vi "Functaion Air Temperature to Density.vi"(5 "Temp(F)":dbl) -> (6 "Density (lb/ft3)":dbl)   [LabVIEW 2012]
uses:
  <vilib>/gmath/NI_Gmath.lvlib
panel:
  in  "Density":dbl[](array[numeric])=[0.081, 0.08, 0.0766, 0.073, 0.0717, 0.071, 0.0698, 0.0692, 0.0685, 0.0674, 0.0662, 0.0651, 0.064, 0.063, 0.062, 0.061, 0.0601, 0.0592, 0.057, 0.055, 0.0531, 0.0513]
  in  "Temps":dbl[](array[numeric])=[30.0, 40.0, 50.0, 75.0, 85.0, 95.0, 100.0, 105.0, 110.0, 120.0, 130.0, 140.0, 150.0, 160.0, 170.0, 180.0, 190.0, 200.0, 225.0, 250.0, 275.0, 300.0]
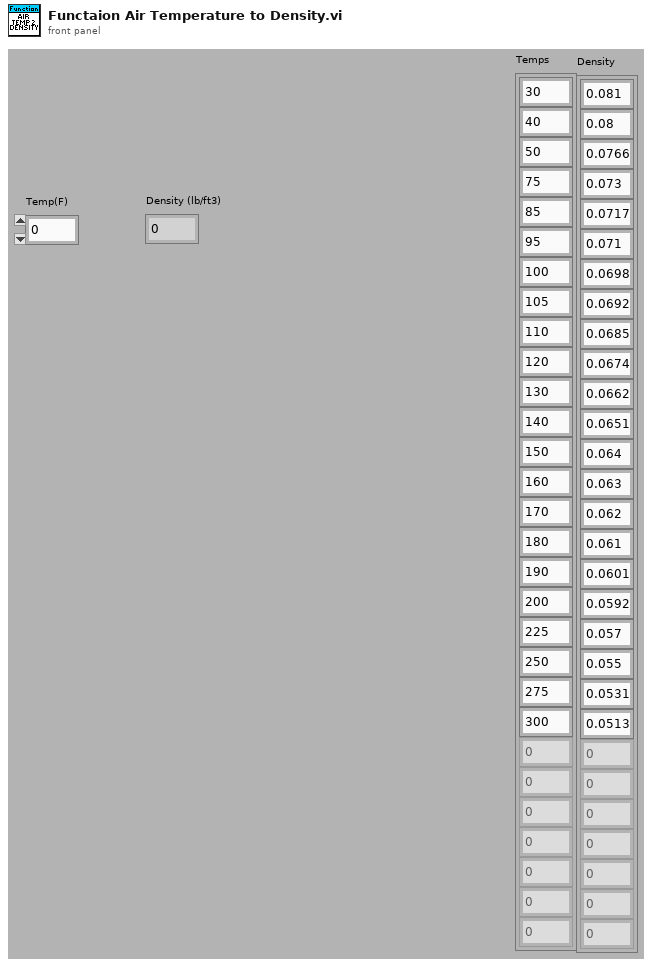
[diagram p1: front panel]
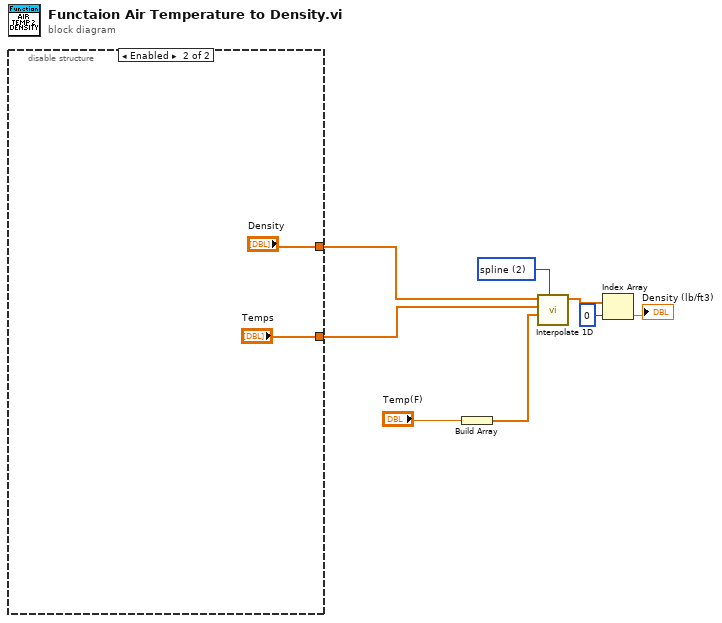
[diagram p0: block diagram]
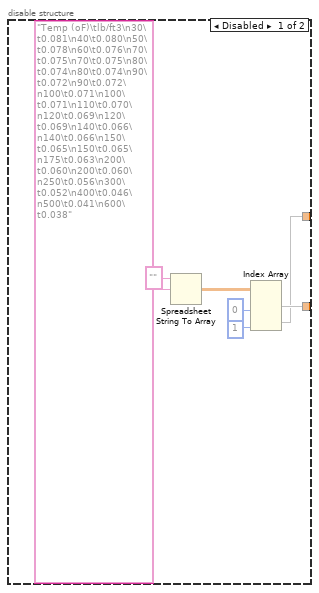
[diagram p2: hidden frame]
diagram:
  w8 = 2 items=["nearest", "linear", "spline", "cubic Hermite", "Lagrange"] ("method")
  n1 = disable-structure shown="Enabled" {
    disable-tunnel: [w10 "Temps"] -> w7
    disable-tunnel: [w9 "Density"] -> w6
    frame Disabled {
      n2 = Spreadsheet String To Array(format string="", spreadsheet string="Temp (oF)\tlb/ft3\n30\t0.081\n40\t0.080\n50\t0.078\n60\t0.076\n70\t0.075\n70\t0.075\n80\t0.074\n80\t0.074\n90\t0.072\n90\t0.072\n100\t0.071\n100\t0.071\n110\t0.070\n120\t0.069\n120\t0.069\n140\t0.066\n140\t0.066\n150\t0.065\n150\t0.065\n175\t0.063\n200\t0.060\n200\t0.060\n250\t0.056\n300\t0.052\n400\t0.046\n500\t0.041\n600\t0.038") -> (array=w13:dbl[][])  [unwired: 2 in]
      n3 = Index Array(array=w13, index (col) #1=0 ("disabled index (col)"), index (col) #2=1 ("index (col)")) -> (element #1=w10:dbl[], element #2=w9:dbl[])  [unwired: 2 in]
    }
    frame Enabled {
    }
  }
  n4 = Build Array("Temp(F)") -> (w4:dbl[])
  n5 = call <vilib>:"Interpolate 1D.vi"("method"=w8, "xi"=w4, "X"=w7, "Y"=w6) -> ("yi"=w5:dbl[])  [unwired: 5 in, 2 out]
  n6 = Index Array(array=w5, index=0) -> (element=→"Density (lb/ft3)":dbl)
